vi "Get Parameter Name.vi"(8 "error in":errorcluster, 11 "Sub Object in":refnum<class "Sub Object.lvclass">) -> (0 "error out":errorcluster, 2 "Parameter Name":string, 3 "Sub Object out":refnum<class "Sub Object.lvclass">)   [LabVIEW 2020, in "CANopen.lvlib" / "Sub Object.lvclass"]
uses:
  Sub Object.lvclass
  Sub Object.lvclass/Sub Object.ctl
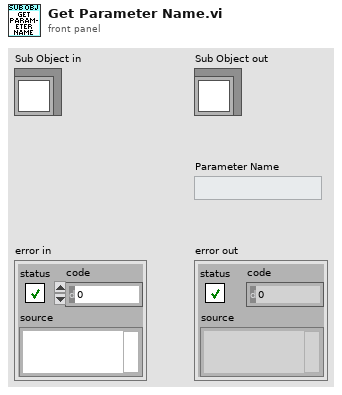
[diagram p1: front panel]
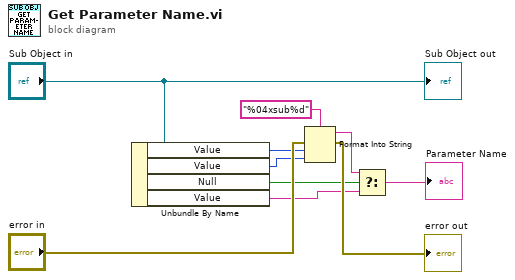
[diagram p0: block diagram]
diagram:
  n1 = Unbundle By Name("Sub Object in") -> ("Value"=w3:u16, "Value"=w4:u8, "Null"=w6:bool, "Value"=w5:string)
  n2 = Format Into String(format string="%04xsub%d", error in="error in", w3, w4) -> (resulting string=w1:string, error out=→"error out":errorcluster)  [unwired: 1 in]
  n3 = Select(t=w1, s=w6, f=w5) -> (s? t:f=→"Parameter Name":string)
  "Sub Object out" <- "Sub Object in"
